vi "act_19-MM.vi"() -> ()   [LabVIEW 2010]
uses:
  act/lv_07/lv_07.lvlib
panel:
  out "Te":dbl
  in  "Cc":dbl
  in  "T":dbl
  out "error out":errorcluster caption="err out"
  in  "error in":errorcluster caption="err in"
  out "Qe":dbl
  in  "Pu":dbl
  in  "Qa":dbl
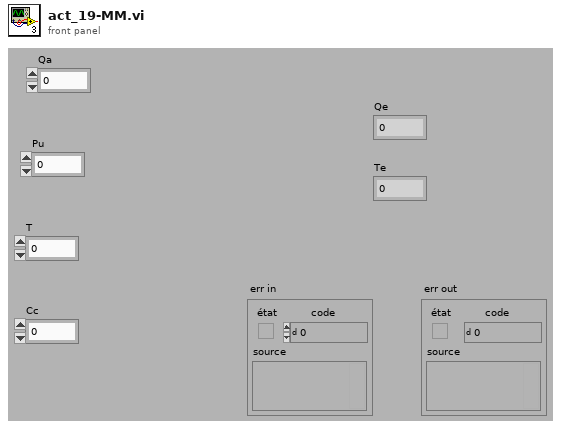
[diagram p1: front panel]
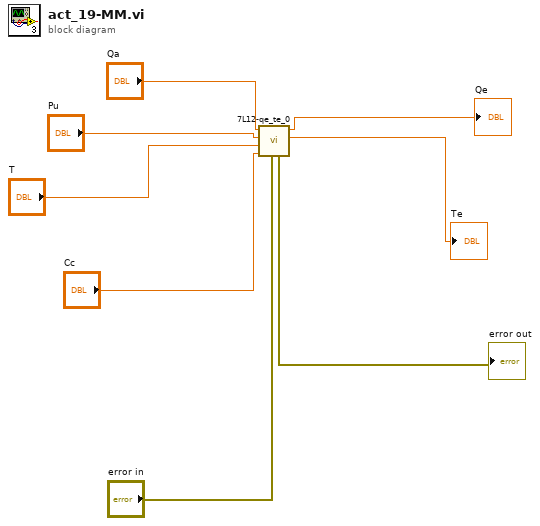
[diagram p0: block diagram]
diagram:
  n1 = call "7L12-qe_te_0.vi"("err in"="error in", "Cc"="Cc", "T"="T", "Pu"="Pu", "Qa"="Qa") -> ("Te (en mois)"=→"Te":dbl, "Qe"=→"Qe":dbl, "error out"=→"error out":errorcluster)  [unwired: 4 in]
